vi "read chart.vi"(4 "file name (.txt)":string) -> (0 "note count":i32, 1 "song info":T1)   [LabVIEW 2023]
uses:
  <vilib>/Utility/error.llb/Trim Whitespace One-Sided.vi
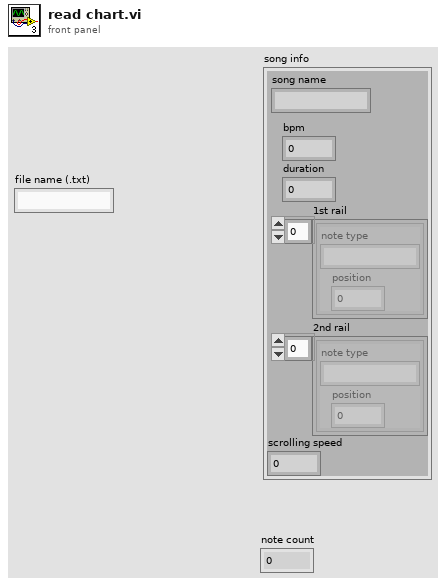
[diagram p1: front panel]
types:
  T1 = cluster{"song name":string, "bpm":i32, "duration":i32, "1st rail":cluster{"note type":string, "position":dbl}[], "2nd rail":cluster{"note type":string, "position":dbl}[], "scrolling speed":dbl}
  T2 = cluster{"String":string, i32, i32, "1st rail":cluster{"note type":string, "position":dbl}[], "2nd rail":cluster{"note type":string, "position":dbl}[], dbl}
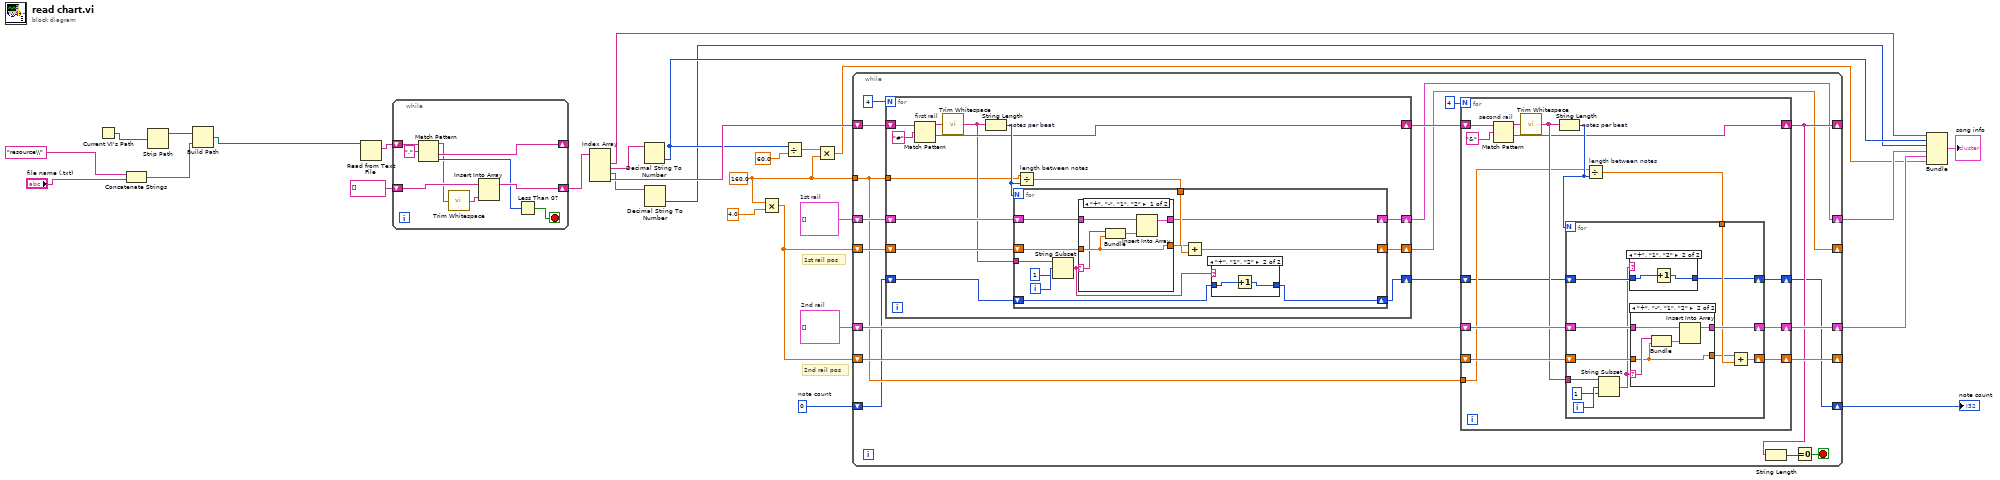
[diagram p0: block diagram]
diagram:
  w8 = 0  # note count
  w14 = 160.0
  w23 = cluster{"note type":string, "position":dbl}[] []  # 2nd rail
  w24 = cluster{"note type":string, "position":dbl}[] []  # 1st rail
  # "2nd rail pos"
  # "1st rail pos"
  n1 = Current VI's Path() -> (path=w6:path)
  n2 = Concatenate Strings("resource\\" ("string"), "file name (.txt)") -> (w2:string)
  n3 = Strip Path(path=w6) -> (stripped path=w5:path)  [unwired: 1 out]
  n4 = Build Path(base path=w5, name or relative path=w2) -> (appended path=w1:path)
  n5 = Read from Text File(file (use dialog)=w1) -> (text=w27:string)  [unwired: 3 in, 3 out]
  n6 = while {
    shift-right: [w33] -> w26
    shift-left: string[] [] -> [w34]
    shift-right: [w35] -> _
    shift-left: w27 -> [w37]
    stop <- w31 stop-if-true
    n7 = Match Pattern(string=w37, regular expression=",") -> (before substring=w30:string, after substring=w35:string, offset past match=w32:i32)  [unwired: 1 in, 1 out]
    n8 = call <vilib>:"Trim Whitespace.vi"("string"=w30) -> ("trimmed string"=w29:string)  [unwired: 1 in]
    n9 = Insert Into Array(array=w34, new element=w29) -> (w33:string[])  [unwired: 1 in]
    n10 = Less Than 0?(x=w32) -> (x < 0?=w31:bool)
  }
  n11 = Index Array(array=w26) -> (element #1=w18:string, element #2=w25:string, element #3=w19:string, element #4=w20:string)  [unwired: 4 in]
  n12 = Decimal String To Number(string=w25) -> (number=w17:i32)  [unwired: 2 in, 1 out]
  n13 = Decimal String To Number(string=w19) -> (number=w16:i32)  [unwired: 2 in, 1 out]
  n14 = Multiply(x=w14, y=4.0) -> (x*y=w12:dbl)
  n15 = Divide(x=w17, y=60.0) -> (x/y=w11:dbl)
  n16 = Multiply(x=w11, y=w14) -> (x*y=w9:dbl)
  n17 = while {
    shift-right: [w44] -> _
    shift-left: w20 -> [w56]
    shift-right: [w42] -> w22
    shift-left: w24 -> [w55]
    shift-right: [w48] -> w21
    shift-left: w23 -> [w50]
    shift-right: [w43] -> _
    shift-left: w12 -> [w54]
    shift-right: [w47] -> _
    shift-left: w12 -> [w49]
    tunnel: w14 -> [w46]
    shift-right: [w38] -> w7
    shift-left: w8 -> [w40]
    stop <- w51 stop-if-true
    n18 = for {
      N: 4 -> [_]
      tunnel: w46 -> [w95]
      shift-right: [w98] -> w53
      shift-left: w56 -> [w106]
      shift-right: [w100] -> w43
      shift-left: w54 -> [w101]
      shift-right: [w99] -> w42
      shift-left: w55 -> [w102]
      shift-right: [w93] -> w39
      shift-left: w40 -> [w94]
      n19 = Match Pattern "first rail"(string=w106, regular expression="#") -> (before substring=w97:string, after substring=w98:string)  [unwired: 1 in, 2 out]
      n20 = call <vilib>:"Trim Whitespace.vi"("string"=w97) -> ("trimmed string"=w96:string)  [unwired: 1 in]
      n21 = String Length "notes per beat"(string=w96) -> (length=w104:i32)
      n22 = Divide "length between notes"(x=w95, y=w104) -> (x/y=w103:dbl)
      n23 = for {
        N: w104 -> [_]
        tunnel: w96 -> [w118]
        tunnel: w103 -> [w111]
        shift-right: [w114] -> w100
        shift-left: w101 -> [w113]
        shift-right: [w110] -> w99
        shift-left: w102 -> [w115]
        shift-right: [w107] -> w93
        shift-left: w94 -> [w108]
        i -> [w117]
        n24 = String Subset(string=w118, offset (0)=w117, length (rest)=1 ("length (rest)")) -> (substring=w109:string)
        n25 = case shown="\"+\", \"-\", \"1\", \"2\"" w109 {
          selector: w109 -> [w122 _]
          tunnel: w115 -> [w126 w127]
          tunnel: w113 -> [w123 w128]
          tunnel: [w123 w128] -> w112
          tunnel: [w125 w127] -> w110
          frame "+", "-", "1", "2" {
            n26 = Bundle(w122, w123) -> (w124:cluster{string, dbl})  [unwired: 1 in]
            n27 = Insert Into Array(array=w126, new element=w124) -> (w125:cluster{"note type":string, "position":dbl}[])  [unwired: 1 in]
          }
          frame "0", Default {
          }
        }
        n28 = Add(x=w111, y=w112) -> (x+y=w114:dbl)
        n29 = case shown="\"+\", \"1\", \"2\"" w109 {
          tunnel: w108 -> [w119 w121]
          tunnel: [w119 w120] -> w107
          frame Default {
          }
          frame "+", "1", "2" {
            n30 = Increment(x=w121) -> (x+1=w120:i32)
          }
        }
      }
    }
    n31 = for {
      N: 4 -> [_]
      tunnel: w46 -> [w60]
      shift-right: [w59] -> w44
      shift-left: w53 -> [w70]
      shift-right: [w66] -> w48
      shift-left: w50 -> [w68]
      shift-right: [w65] -> w47
      shift-left: w49 -> [w67]
      shift-right: [w57] -> w38
      shift-left: w39 -> [w58]
      n32 = Match Pattern "second rail"(string=w70, regular expression="&") -> (before substring=w62:string, after substring=w59:string)  [unwired: 1 in, 2 out]
      n33 = call <vilib>:"Trim Whitespace.vi"("string"=w62) -> ("trimmed string"=w61:string)  [unwired: 1 in]
      n34 = String Length "notes per beat"(string=w61) -> (length=w63:i32)
      n35 = Divide "length between notes"(x=w60, y=w63) -> (x/y=w64:dbl)
      n36 = for {
        N: w63 -> [_]
        tunnel: w61 -> [w81]
        shift-right: [w78] -> w66
        shift-left: w68 -> [w79]
        shift-right: [w77] -> w65
        shift-left: w67 -> [w75]
        tunnel: w64 -> [w76]
        shift-right: [w71] -> w57
        shift-left: w58 -> [w73]
        i -> [w82]
        n37 = String Subset(string=w81, offset (0)=w82, length (rest)=1 ("length (rest)")) -> (substring=w72:string)
        n38 = case shown="\"+\", \"1\", \"2\"" w72 {
          tunnel: w73 -> [w83 w85]
          tunnel: [w83 w84] -> w71
          frame Default {
          }
          frame "+", "1", "2" {
            n39 = Increment(x=w85) -> (x+1=w84:i32)
          }
        }
        n40 = case shown="\"+\", \"-\", \"1\", \"2\"" w72 {
          selector: w72 -> [_ w89]
          tunnel: w79 -> [w87 w92]
          tunnel: [w87 w91] -> w78
          tunnel: w75 -> [w86 w88]
          tunnel: [w86 w88] -> w74
          frame "0", Default {
          }
          frame "+", "-", "1", "2" {
            n41 = Bundle(w89, w88) -> (w90:cluster{string, dbl})  [unwired: 1 in]
            n42 = Insert Into Array(array=w92, new element=w90) -> (w91:cluster{"note type":string, "position":dbl}[])  [unwired: 1 in]
          }
        }
        n43 = Add(x=w74, y=w76) -> (x+y=w77:dbl)
      }
    }
    n44 = String Length(string=w44) -> (length=w52:i32)
    n45 = Equal To 0?(x=w52) -> (x = 0?=w51:bool)
  }
  "note count" <- w7
  n46 = Bundle("String"=w18, w17, w16, "1st rail"=w22, "2nd rail"=w21, w9) -> (→"song info":T2)  [unwired: 1 in]
